vi "Git-Convert git Timestamp to Timestamp.vi"(5 "Git Timestamp":string="2020-06-22T02:35:28Z") -> (2 "Time Stamp":timestamp)   [LabVIEW 2020]
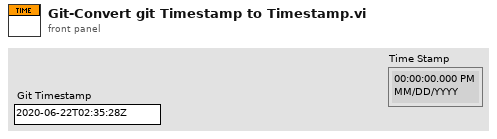
[diagram p1: front panel]
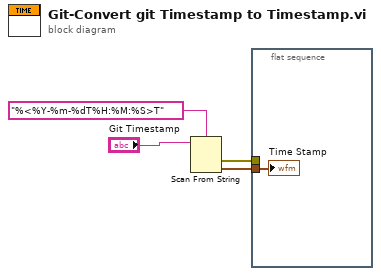
[diagram p0: block diagram]
diagram:
  n1 = Scan From String(format string="%<%Y-%m-%dT%H:%M:%S>T", input string="Git Timestamp") -> (error out=w1:errorcluster, output 1=w2:timestamp)  [unwired: 3 in, 2 out]
  n2 = flat-sequence {
    tunnel: w2 -> [w5]
    tunnel: w1 -> [_]
    frame #0 {
      "Time Stamp" <- w5
    }
  }
